vi "Module_SMU_Measurements.vi"(8 "Error In":errorcluster, 11 "Instrument_Visas":T1) -> (0 "Error Out":errorcluster, 1 "Throw_Resitances":dbl[](array[numeric]) format="%#_6p", 2 "Throw Measurements":T2 {"current measurements" format="%#_6p"}, 3 "Dut and Bridge Measurements":T2 {"current measurements" format="%#_6p"})   [LabVIEW 2013]
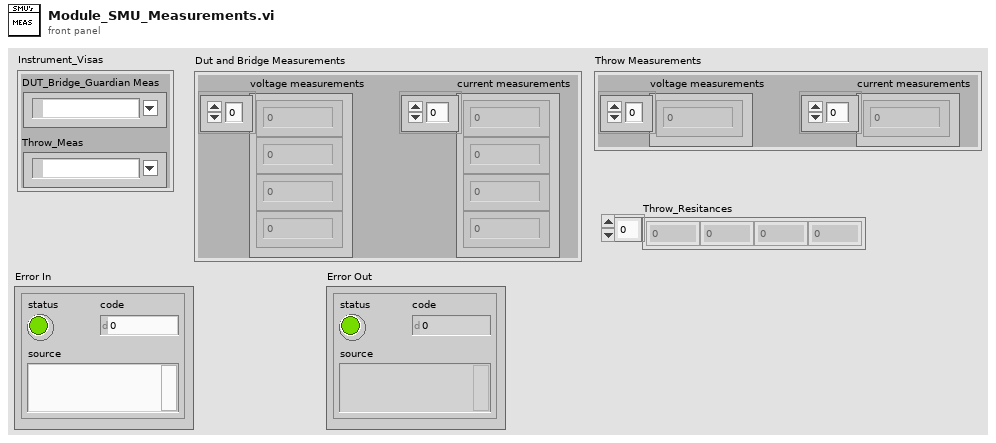
[diagram p1: front panel]
types:
  T1 = cluster{"DUT_Bridge_Guardian Meas":refnum<k15>, "Throw_Meas":refnum<k15>}
  T2 = cluster{"voltage measurements":dbl[], "current measurements":dbl[]}
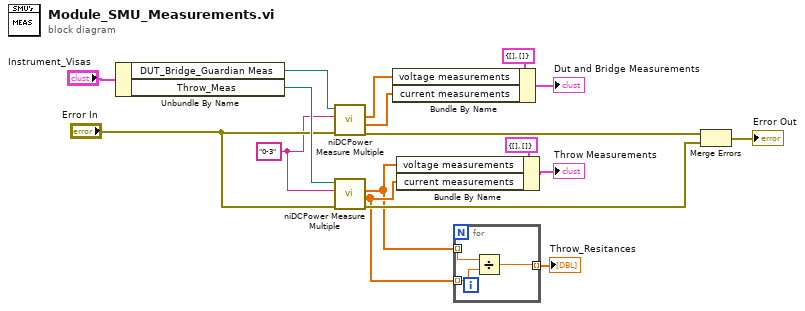
[diagram p0: block diagram]
diagram:
  w5 = "0-3" ("channel name")
  n1 = Unbundle By Name("Instrument_Visas") -> ("DUT_Bridge_Guardian Meas"=w17:refnum<k15>, "Throw_Meas"=w16:refnum<k15>)
  n2 = call <instrlib>:"niDCPower Measure Multiple.vi"("error in (no error)"="Error In", "channel name"=w5, "instrument handle"=w17) -> ("error out"=w8:errorcluster, "current measurements"=w13:dbl[], "voltage measurements"=w14:dbl[])  [unwired: 5 in, 1 out]
  n3 = call <instrlib>:"niDCPower Measure Multiple.vi"("error in (no error)"="Error In", "channel name"=w5, "instrument handle"=w16) -> ("error out"=w4:errorcluster, "current measurements"=w3:dbl[], "voltage measurements"=w2:dbl[])  [unwired: 5 in, 1 out]
  n4 = Bundle By Name(cluster=T2 {"voltage measurements"=[], "current measurements"=[]} ("Dut and Bridge Measurements"), "voltage measurements"=w14, "current measurements"=w13) -> (→"Dut and Bridge Measurements":T2)
  n5 = Bundle By Name(cluster=T2 {"voltage measurements"=[], "current measurements"=[]} ("Dut and Bridge Measurements"), "voltage measurements"=w2, "current measurements"=w3) -> (→"Throw Measurements":T2)
  n6 = for {
    tunnel: w3 -> [w19] mode=indexing
    tunnel: w2 -> [w20] mode=indexing
    tunnel: [w18] -> w1 mode=indexing
    n7 = Divide(x=w20, y=w19) -> (x/y=w18:dbl)
  }
  "Throw_Resitances" <- w1
  n8 = Merge Errors(w8, w4) -> (→"Error Out":errorcluster)
